vi "read TDMS.vi"   [LabVIEW 2015]
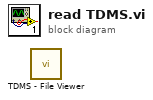
[diagram p0: block diagram]
diagram:
  n1 = call <vilib>:"TDMS - File Viewer.vi"() -> ()  [unwired: 6 in, 2 out]
